vi "to_xml.vi"(8 "error in":errorcluster, 11 "Analog Output Parameters":T1={"Enable Analog Out?"=FALSE, "Physical Channel"="PXI1Slot2/ao0:2", "Minimum Value"=-10.0, "Maximum Value"=10.0, "Samples per second"=0.0, "Total AO Time (seconds)"=0.0, "Start Trigger"={"Wait for start trigger?"=FALSE, "source"="/Dev1/PFI0", "edge"=10280}, "Analog Output Waveforms (channel, time)"=[], "Export trigger"={"Export Start Trigger?"=FALSE, "output terminal"=""}} {"Start Trigger"."edge" items=["Rising"=10280, "Falling"=10171]; "Maximum Value" format="%0.2f"; "Minimum Value" format="%0.2f"}) -> (0 "error out":errorcluster, 3 "Analog Output Settings string":string)   [LabVIEW 2013, in "Analog_Output.lvclass"]
doc: "Saves analog output settings into xml in the format:\n\n<Enable>%b</Enable>\n<PhysicalChannel>%s</PhysicalChannel>\n<MinimumValue>%f</MinimumValue>\n<MaximumValue>%f</MaximumValue>\n<SamplesPerSecond>%f</SamplesPerSecond>\n<TotalAOTime units=\"seconds\">%s</TotalAOTime>\n<AnalogOutputEquations>\n%s</AnalogOutputEquations>\n<StartTrigger.WaitForStartTrigger>%b</StartTrigger.WaitForStartTrigger\n<StartTrigger.source>%s</StartTrigger.source>\n<StartTrigger.edge>%s</StartTrigger.edge>\n\nMTL 2012 Dec 31"
uses:
  Analog_Output.lvclass
  AO_settings.ctl
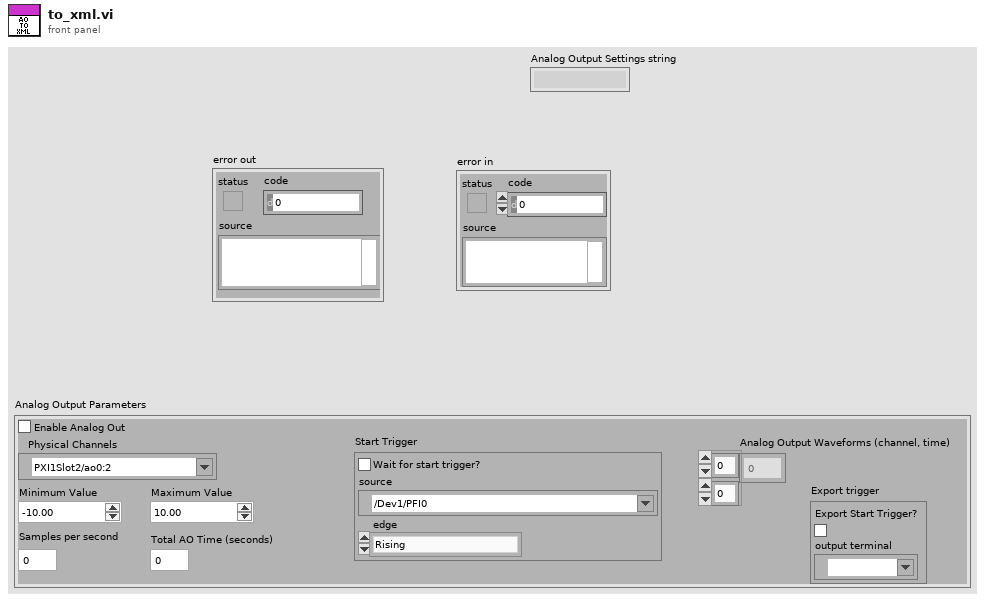
[diagram p1: front panel]
types:
  T1 = typedef "Analog_Output.lvclass/AO_settings.ctl" = cluster{"Enable Analog Out?":bool, "Physical Channel":tag, "Minimum Value":dbl, "Maximum Value":dbl, "Samples per second":dbl, "Total AO Time (seconds)":dbl, "Start Trigger":cluster{"Wait for start trigger?":bool, "source":tag, "edge":i32}, "Analog Output Waveforms (channel, time)":dbl[][], "Export trigger":cluster{"Export Start Trigger?":bool, "output terminal":tag}}
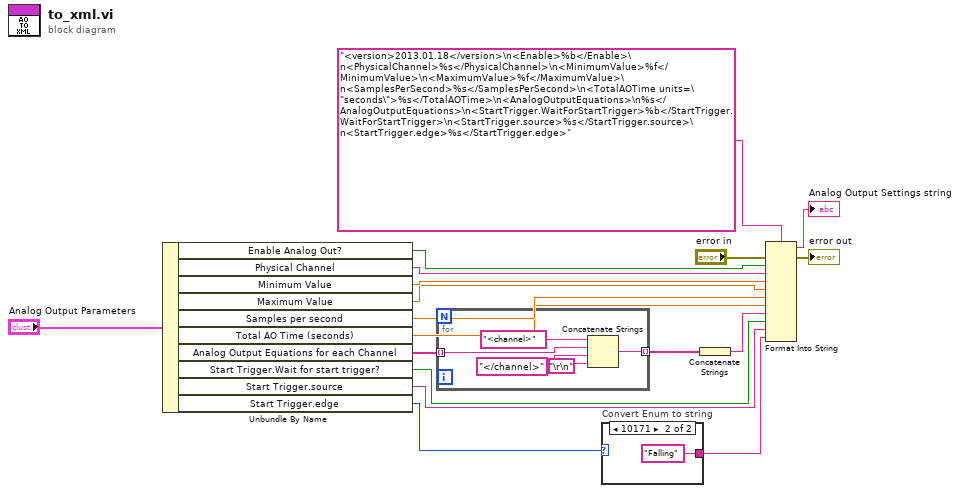
[diagram p0: block diagram]
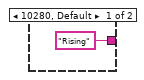
[diagram p2: hidden frame]
diagram:
  n1 = Unbundle By Name("Analog Output Parameters") -> ("Enable Analog Out?"=w17:bool, "Physical Channel"=w16:tag, "Minimum Value"=w15:dbl, "Maximum Value"=w14:dbl, "Samples per second"=w13:dbl, "Total AO Time (seconds)"=w12:dbl, "Analog Output Equations for each Channel"=w9:string[], "Start Trigger.Wait for start trigger?"=w11:bool, "Start Trigger.source"=w10:tag, "Start Trigger.edge"=w2:i32)
  n2 = for {
    tunnel: w9 -> [w21] mode=indexing
    tunnel: [w23] -> w4 mode=indexing
    n3 = Concatenate Strings("<channel>" ("string"), w21, "</channel>" ("string"), "\r\n") -> (w23:string)
  }
  n4 = case "Convert Enum to string" shown="10171" w2 {
    tunnel: ["Rising" ("string") "Falling" ("string")] -> w1
    frame 10280, Default {
    }
    frame 10171 {
    }
  }
  n5 = Concatenate Strings(w4) -> (w3:string)
  n6 = Format Into String(format string="<version>2013.01.18</version>\n<Enable>%b</Enable>\n<PhysicalChannel>%s</PhysicalChannel>\n<MinimumValue>%f</MinimumValue>\n<MaximumValue>%f</MaximumValue>\n<SamplesPerSecond>%s</SamplesPerSecond>\n<TotalAOTime units=\"seconds\">%s</TotalAOTime>\n<AnalogOutputEquations>\n%s</AnalogOutputEquations>\n<StartTrigger.WaitForStartTrigger>%b</StartTrigger.WaitForStartTrigger>\n<StartTrigger.source>%s</StartTrigger.source>\n<StartTrigger.edge>%s</StartTrigger.edge>", error in="error in", w17, w16, w15, w14, w13, w12, w3, w11, w10, w1) -> (resulting string=→"Analog Output Settings string":string, error out=→"error out":errorcluster)  [unwired: 1 in]
